vi "ROICenter2LTRB.vi"(2 "error out 3":errorcluster, 3 "Selected array":dbl[][](array[numeric]), 4 "ROI (pix)":i32) -> (0 "error out 2":errorcluster, 1 "Array":dbl[][](array[numeric]))   [LabVIEW 2011]
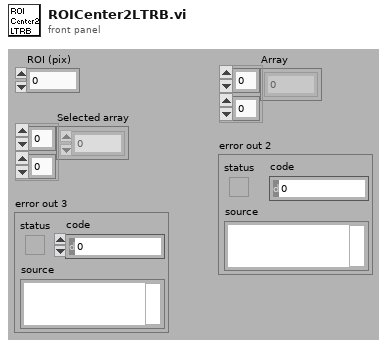
[diagram p1: front panel]
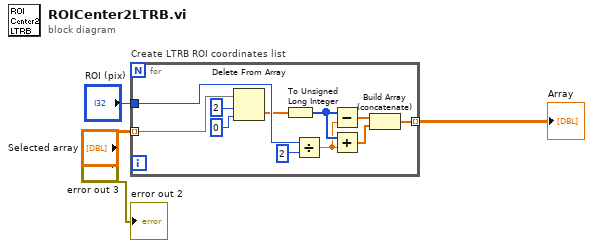
[diagram p0: block diagram]
diagram:
  n1 = for "Create LTRB ROI coordinates list" {
    tunnel: "ROI (pix)" -> [w14]
    tunnel: "Selected array" -> [w15] mode=indexing
    tunnel: [w8] -> w4 mode=indexing
    n2 = Delete From Array(array=w15, length=2, index=0) -> (deleted portion=w13:dbl[])  [unwired: 1 out]
    n3 = To Unsigned Long Integer(number=w13) -> (unsigned 32bit integer=w7:u32[])
    n4 = Divide(x=w14, y=2) -> (x/y=w6:dbl)
    n5 = Subtract(x=w7, y=w6) -> (x-y=w10:dbl[])
    n6 = Add(x=w7, y=w6) -> (x+y=w9:dbl[])
    n7 = Build Array (concatenate)(w10, w9) -> (w8:dbl[])
  }
  "Array" <- w4
  "error out 2" <- "error out 3"
